vi "Read Measurement Times.vi"(8 "error in (no error)":errorcluster, 11 "ModeSwitch Eval in":refnum<class "ModeSwitch Eval.lvclass">) -> (0 "error out":errorcluster, 2 "Measurement Times":string[](array[string]), 3 "ModeSwitch Eval out":refnum<class "ModeSwitch Eval.lvclass">)   [LabVIEW 2016, in "SeqAuto Evaluations.lvlib" / "ModeSwitch Eval.lvclass"]
uses:
  ModeSwitch Eval.lvclass
  ModeSwitch Eval.lvclass/ModeSwitch Eval.ctl
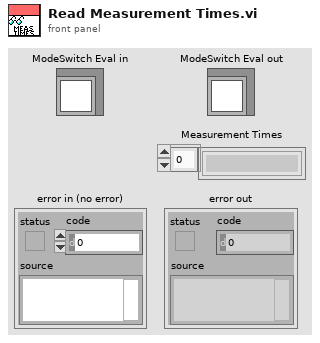
[diagram p1: front panel]
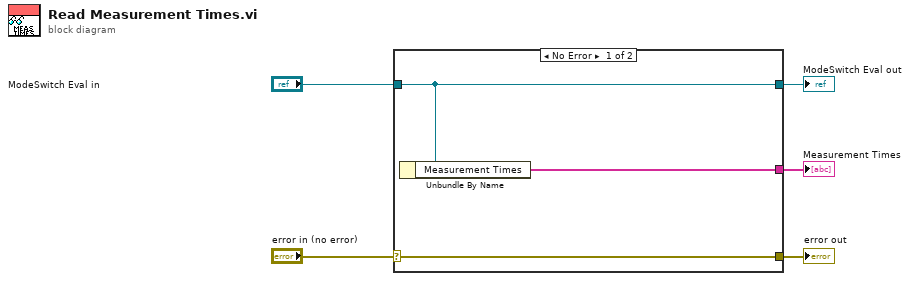
[diagram p0: block diagram]
diagram:
  n1 = case shown="No Error" "error in (no error)" {
    selector: "error in (no error)" -> [w8 w9]
    tunnel: [w8 w9] -> w4
    tunnel: [w7 w10] -> w2
    tunnel: "ModeSwitch Eval in" -> [w7 w10]
    tunnel: [w6 _] -> w1
    frame No Error {
      n2 = Unbundle By Name(w7) -> ("Measurement Times"=w6:string[])
    }
    frame Error {
    }
  }
  "error out" <- w4
  "ModeSwitch Eval out" <- w2
  "Measurement Times" <- w1
